vi "Create New Tag Names.vi"(2 "Prefix":string, 3 "N0":dbl, 4 "N task":dbl) -> (0 "Filename":string)   [LabVIEW 2019]
uses:
  <vilib>/Utility/file.llb/Write Delimited Spreadsheet (string).vi
  <vilib>/Utility/file.llb/Read Delimited Spreadsheet (string).vi
panel:
  in  "Last":string[](array[string])
  in  "First":string[](array[string])
  out "all rows":string[][](array[string])
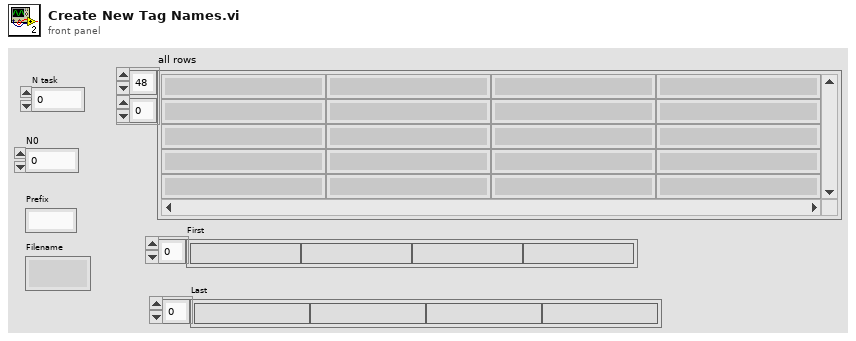
[diagram p1: front panel]
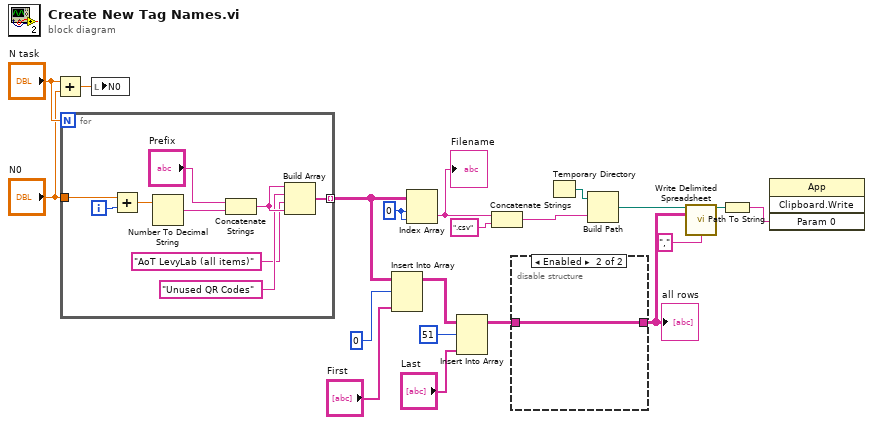
[diagram p0: block diagram]
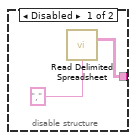
[diagram p2: hidden frame]
diagram:
  w10 = 0 ("index (row)")
  n1 = Add(x="N task", y="N0") -> (x+y=w20:dbl)
  n2 = for {
    N: "N task" -> [_]
    tunnel: "N0" -> [w29]
    tunnel: [w21] -> w11 mode=indexing
    i -> [w28]
    n3 = Add(x=w29, y=w28) -> (x+y=w27:dbl)
    n4 = Number To Decimal String(number=w27) -> (decimal integer string=w26:string)  [unwired: 1 in]
    n5 = Concatenate Strings("Prefix", w26) -> (w24:string)
    n6 = Build Array(w24, "Unused QR Codes" ("element"), "AoT LevyLab (all items)" ("element"), w24) -> (w21:string[])
  }
  n7 = local write "N0"(w20) -> ()
  n8 = Insert Into Array(array=w11, index (row)=0, new element="First") -> (w15:string[][])  [unwired: 1 in]
  n9 = Index Array(array=w11, index (row)=w10, index (col)=w10) -> (element=w8:string)
  "Filename" <- w8
  n10 = Insert Into Array(array=w15, index (row)=51, new element="Last") -> (w12:string[][])  [unwired: 1 in]
  n11 = Concatenate Strings(w8, ".csv" ("string")) -> (w4:string)
  n12 = disable-structure shown="Enabled" {
    disable-tunnel: [w30 w32] -> w9
    disable-tunnel: w12 -> [_ w32]
    frame Disabled {
      n13 = call-poly <vilib>:"Read Delimited Spreadsheet.vi"("delimiter (\\t)"="," ("delimiter (\\t)")) -> ("all rows"=w30:string[][])  [unwired: 9 in, 5 out]
    }
    frame Enabled {
    }
  }
  "all rows" <- w9
  n14 = Temporary Directory() -> (w5:path)
  n15 = Build Path(base path=w5, name or relative path=w4) -> (appended path=w3:path)
  n16 = call-poly <vilib>:"Write Delimited Spreadsheet.vi"("file path (dialog if empty)"=w3, "2D data"=w9, "delimiter (\\t)"="," ("delimiter (\\t)")) -> ("new file path (Not A Path if cancelled)"=w2:path)  [unwired: 11 in, 1 out]
  n17 = Path To String(path=w2) -> (string=w1:string)
  n18 = invoke class="App" method="Clipboard.Write"("Param 0"=w1) -> ()  [unwired: 3 in, 4 out]
